vi "Remove Outliers (Index).vi"(0 "Y":dbl[](array[numeric]), 5 "X":dbl[](array[numeric]), 7 "Weight":dbl[](array[numeric]), 9 "Index":i32[](array[numeric])) -> (4 "Y Out":dbl[](array[numeric]), 6 "X Out":dbl[](array[numeric]), 8 "Weight Out":dbl[](array[numeric]), 15 "error":i32)   [LabVIEW 2018, in "NI_AALPro.lvlib"]
doc: "Removes data points that fall outside a given range or within a given index array. You must manually select the polymorphic instance you want to use."
uses:
  <vilib>/Analysis/NI_AALPro.lvlib
  <resource>/lvanlys.dll
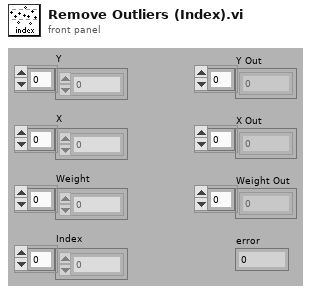
[diagram p1: front panel]
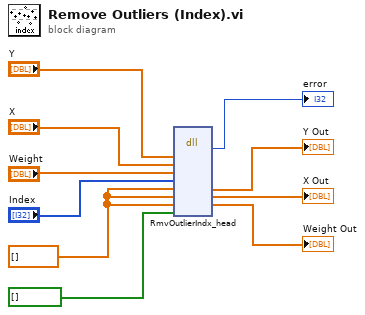
[diagram p0: block diagram]
diagram:
  w1 = dbl[] [] ("Y In")
  n1 = dll-call lib="C:/Program Files (x86)/National Instruments/LabVIEW 2018/resource/lvanlys.*" fn="RmvOutlierIndx_head"("yIn"="Y", "xIn"="X", "wIn"="Weight", "index"="Index", "yOut"=w1, "xOut"=w1, "wOut"=w1, "Outliers"=bool[] []) -> (→"error":i32, "yOut"=→"Y Out":dbl[], "xOut"=→"X Out":dbl[], "wOut"=→"Weight Out":dbl[])  [unwired: 8 in, 2 out]
